vi "Music Element To Music Element Library.vi"(8 "error in (no error)":errorcluster, 11 "MusicElement":refnum<class "MusicElement.lvclass">) -> (0 "error out":errorcluster, 3 "MusicElementLibrary out":refnum<class "MusicElementLibrary.lvclass">)   [LabVIEW 2015, in "MusicElementLibrary.lvclass"]
uses:
  MusicElementLibrary.lvclass
  MusicElement.lvclass
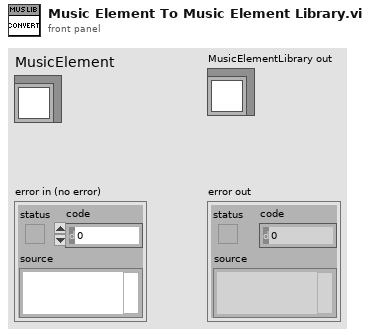
[diagram p1: front panel]
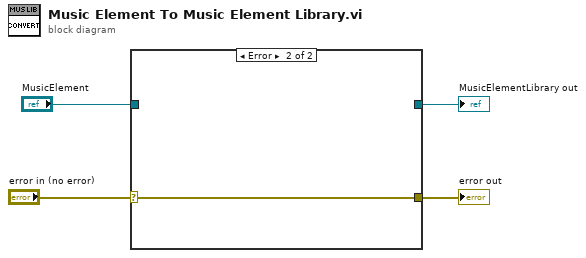
[diagram p0: block diagram]
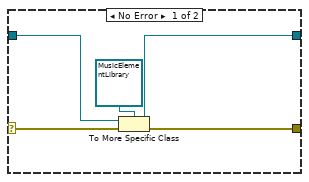
[diagram p2: hidden frame]
diagram:
  n1 = case shown="Error" "error in (no error)" {
    selector: "error in (no error)" -> [w9 w10]
    tunnel: [w5 w10] -> w3
    tunnel: [w6 _] -> w2
    tunnel: "MusicElement" -> [w8 _]
    frame No Error {
      n2 = To More Specific Class(target class=refnum<class "MusicElementLibrary.lvclass"> refnum ("MusicElementLibrary out"), reference=w8, error in=w9) -> (specific class reference=w6:refnum<class "MusicElementLibrary.lvclass">, error out=w5:errorcluster)
    }
    frame Error {
    }
  }
  "error out" <- w3
  "MusicElementLibrary out" <- w2
